vi "getcomport.vi"() -> (0 "No Devices":bool, 1 "Port":string, 4 "Device":string)   [LabVIEW 2012]
uses:
  <vilib>/Instr/_visa.llb/VISA Find Search Mode.ctl
  <vilib>/Utility/error.llb/DialogType.ctl
panel:
  out "Devices":string[](array[string])
  out "Ports":string[](array[string])
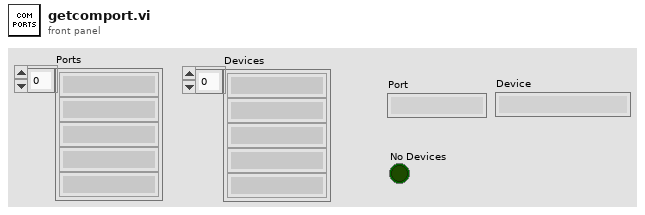
[diagram p1: front panel]
types:
  T1 = typedef "DialogType.ctl" = u16
  T2 = typedef "VISA Find Search Mode.ctl" = u32
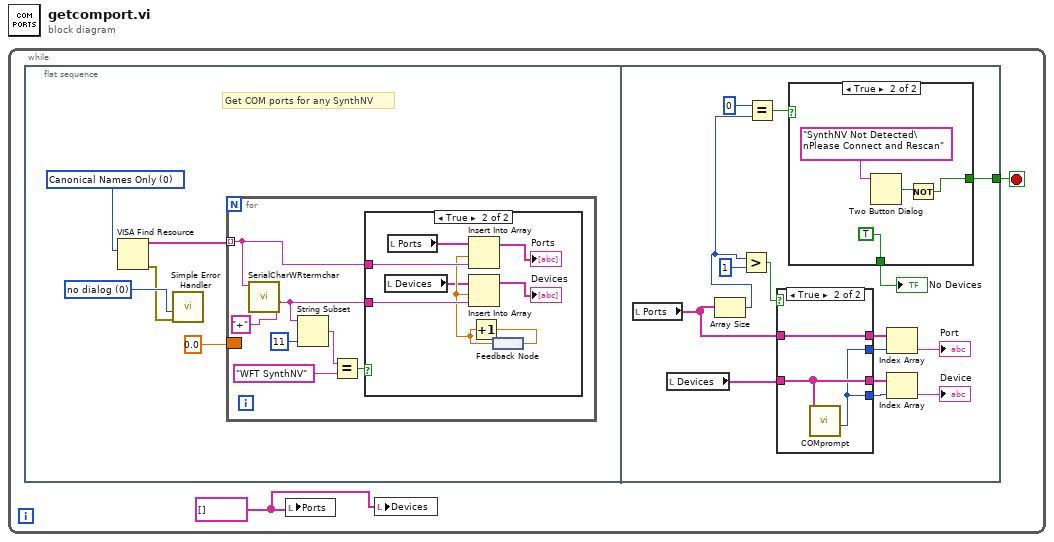
[diagram p0: block diagram]
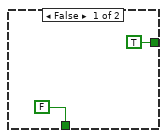
[diagram p3: hidden frame]
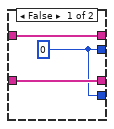
[diagram p4: hidden frame]
diagram:
  n1 = while {
    stop <- w2 stop-if-true
    w1 = string[] [] ("array")
    n2 = flat-sequence {
      tunnel: [w23] -> w2
      frame #0 {
        w6 = T1 0 items=["no dialog", "OK message", "continue or stop message", "OK message + warnings", "continue/stop + warnings"] ("type of dialog (OK msg:1)")
        w7 = T2 0 items=["Canonical Names Only"=0, "Aliases Only"=2, "Include Matching Aliases"=3, "Include All Aliases"=4] ("Search Mode")
        # "Get COM ports for any SynthNV"
        n3 = VISA Find Resource(10:w7) -> (0:w5:errorcluster, 3:w4:string[])  [unwired: 2 in, 1 out]
        n4 = call <vilib>:"Simple Error Handler.vi"("type of dialog (OK msg:1)"=w6, "error in (no error)"=w5) -> ()  [unwired: 8 out]
        n5 = for {
          tunnel: w4 -> [w10] mode=indexing
          border: 0.0 -> [_]
          n6 = call "SerialCharWRtermchar.vi"("VISA resource name"=w10, "write buffer"="+") -> ("read buffer"=w8:string)  [unwired: 6 in, 2 out]
          n7 = String Subset(string=w8, length (rest)=11 ("length (rest)")) -> (substring=w12:string)  [unwired: 1 in]
          n8 = Equal?(x=w12, y="WFT SynthNV") -> (x = y?=w11:bool)
          n9 = case shown="True" w11 {
            tunnel: w8 -> [_ w22]
            tunnel: w10 -> [_ w21]
            frame False {
            }
            frame True {
              n10 = local read "Devices"() -> (w15:string[])
              n11 = local read "Ports"() -> (w16:string[])
              n12 = feedback #1() -> (w17:dbl)
              n13 = Insert Into Array(array=w16, index=w17, new element=w21) -> (→"Ports":string[])
              n14 = Insert Into Array(array=w15, index=w17, new element=w22) -> (→"Devices":string[])
              n15 = Increment(x=w17) -> (x+1=w18:dbl)
              n16 = feedback-in #1(w18) -> ()
            }
          }
        }
      }
      frame #1 {
        n17 = local read "Ports"() -> (w36:string[])
        n18 = local read "Devices"() -> (w37:string[])
        n19 = Array Size(array=w36) -> (size(s)=w33:i32)
        n20 = Greater?(x=w33, y=u32 1) -> (0:w25:bool)
        n21 = Equal?(x=0, y=w33) -> (x = y?=w32:bool)
        n22 = case shown="True" w25 {
          tunnel: w37 -> [w45 w48]
          tunnel: w36 -> [w46 w49]
          tunnel: [w46 w49] -> w27
          tunnel: [w44 w47] -> w28
          tunnel: [w45 w48] -> w29
          tunnel: [w44 w47] -> w30
          frame False {
            w44 = 0 ("Numeric")
          }
          frame True {
            n23 = call "COMprompt.vi"("Devices"=w48) -> ("Numeric"=w47:i32)  [unwired: 10 in]
          }
        }
        n24 = case shown="True" w32 {
          tunnel: [FALSE TRUE] -> w35
          tunnel: [TRUE w40] -> w23
          frame False {
          }
          frame True {
            n25 = Two Button Dialog(message="SynthNV Not Detected\nPlease Connect and Rescan") -> (T button?=w43:bool)  [unwired: 2 in]
            n26 = Not(x=w43) -> (.not. x?=w40:bool)
          }
        }
        "No Devices" <- w35
        n27 = Index Array(array=w27, index=w28) -> (element=→"Port":string)
        n28 = Index Array(array=w29, index=w30) -> (element=→"Device":string)
      }
    }
    n29 = local write "Ports"(w1) -> ()
    n30 = local write "Devices"(w1) -> ()
  }
